vi "TLB Native Dynamic Events ver 0.04.vi"() -> ()   [LabVIEW 2018]
uses:
  Labview Training Phase 2/Enum Controls/States for Action Engine.ctl
  Type def/TLB event states.ctl
panel:
  out "element":T1
  in  "Combo Box":string(combo)
  in  "Stop Queue":bool
  in  "Start Queue":bool
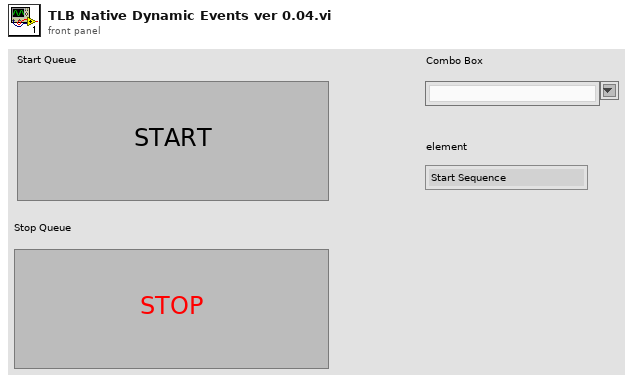
[diagram p1: front panel]
types:
  T1 = typedef "TLB event states.ctl" = enum16{"Start Sequence", "Exit", "Start Task 1", "Start Task 2", "Start Task 3", "Start Task 4", "Camera vision", "Wall follow mode", "Idle", "Start Drive Straight"}
  T2 = typedef "States for Action Engine.ctl" = enum16{"Initialize", "Write", "Read"}
  T3 = typedef "TLB event states.ctl" = enum16{"Start Sequence", "Exit", "Task 1", "Task 2"}
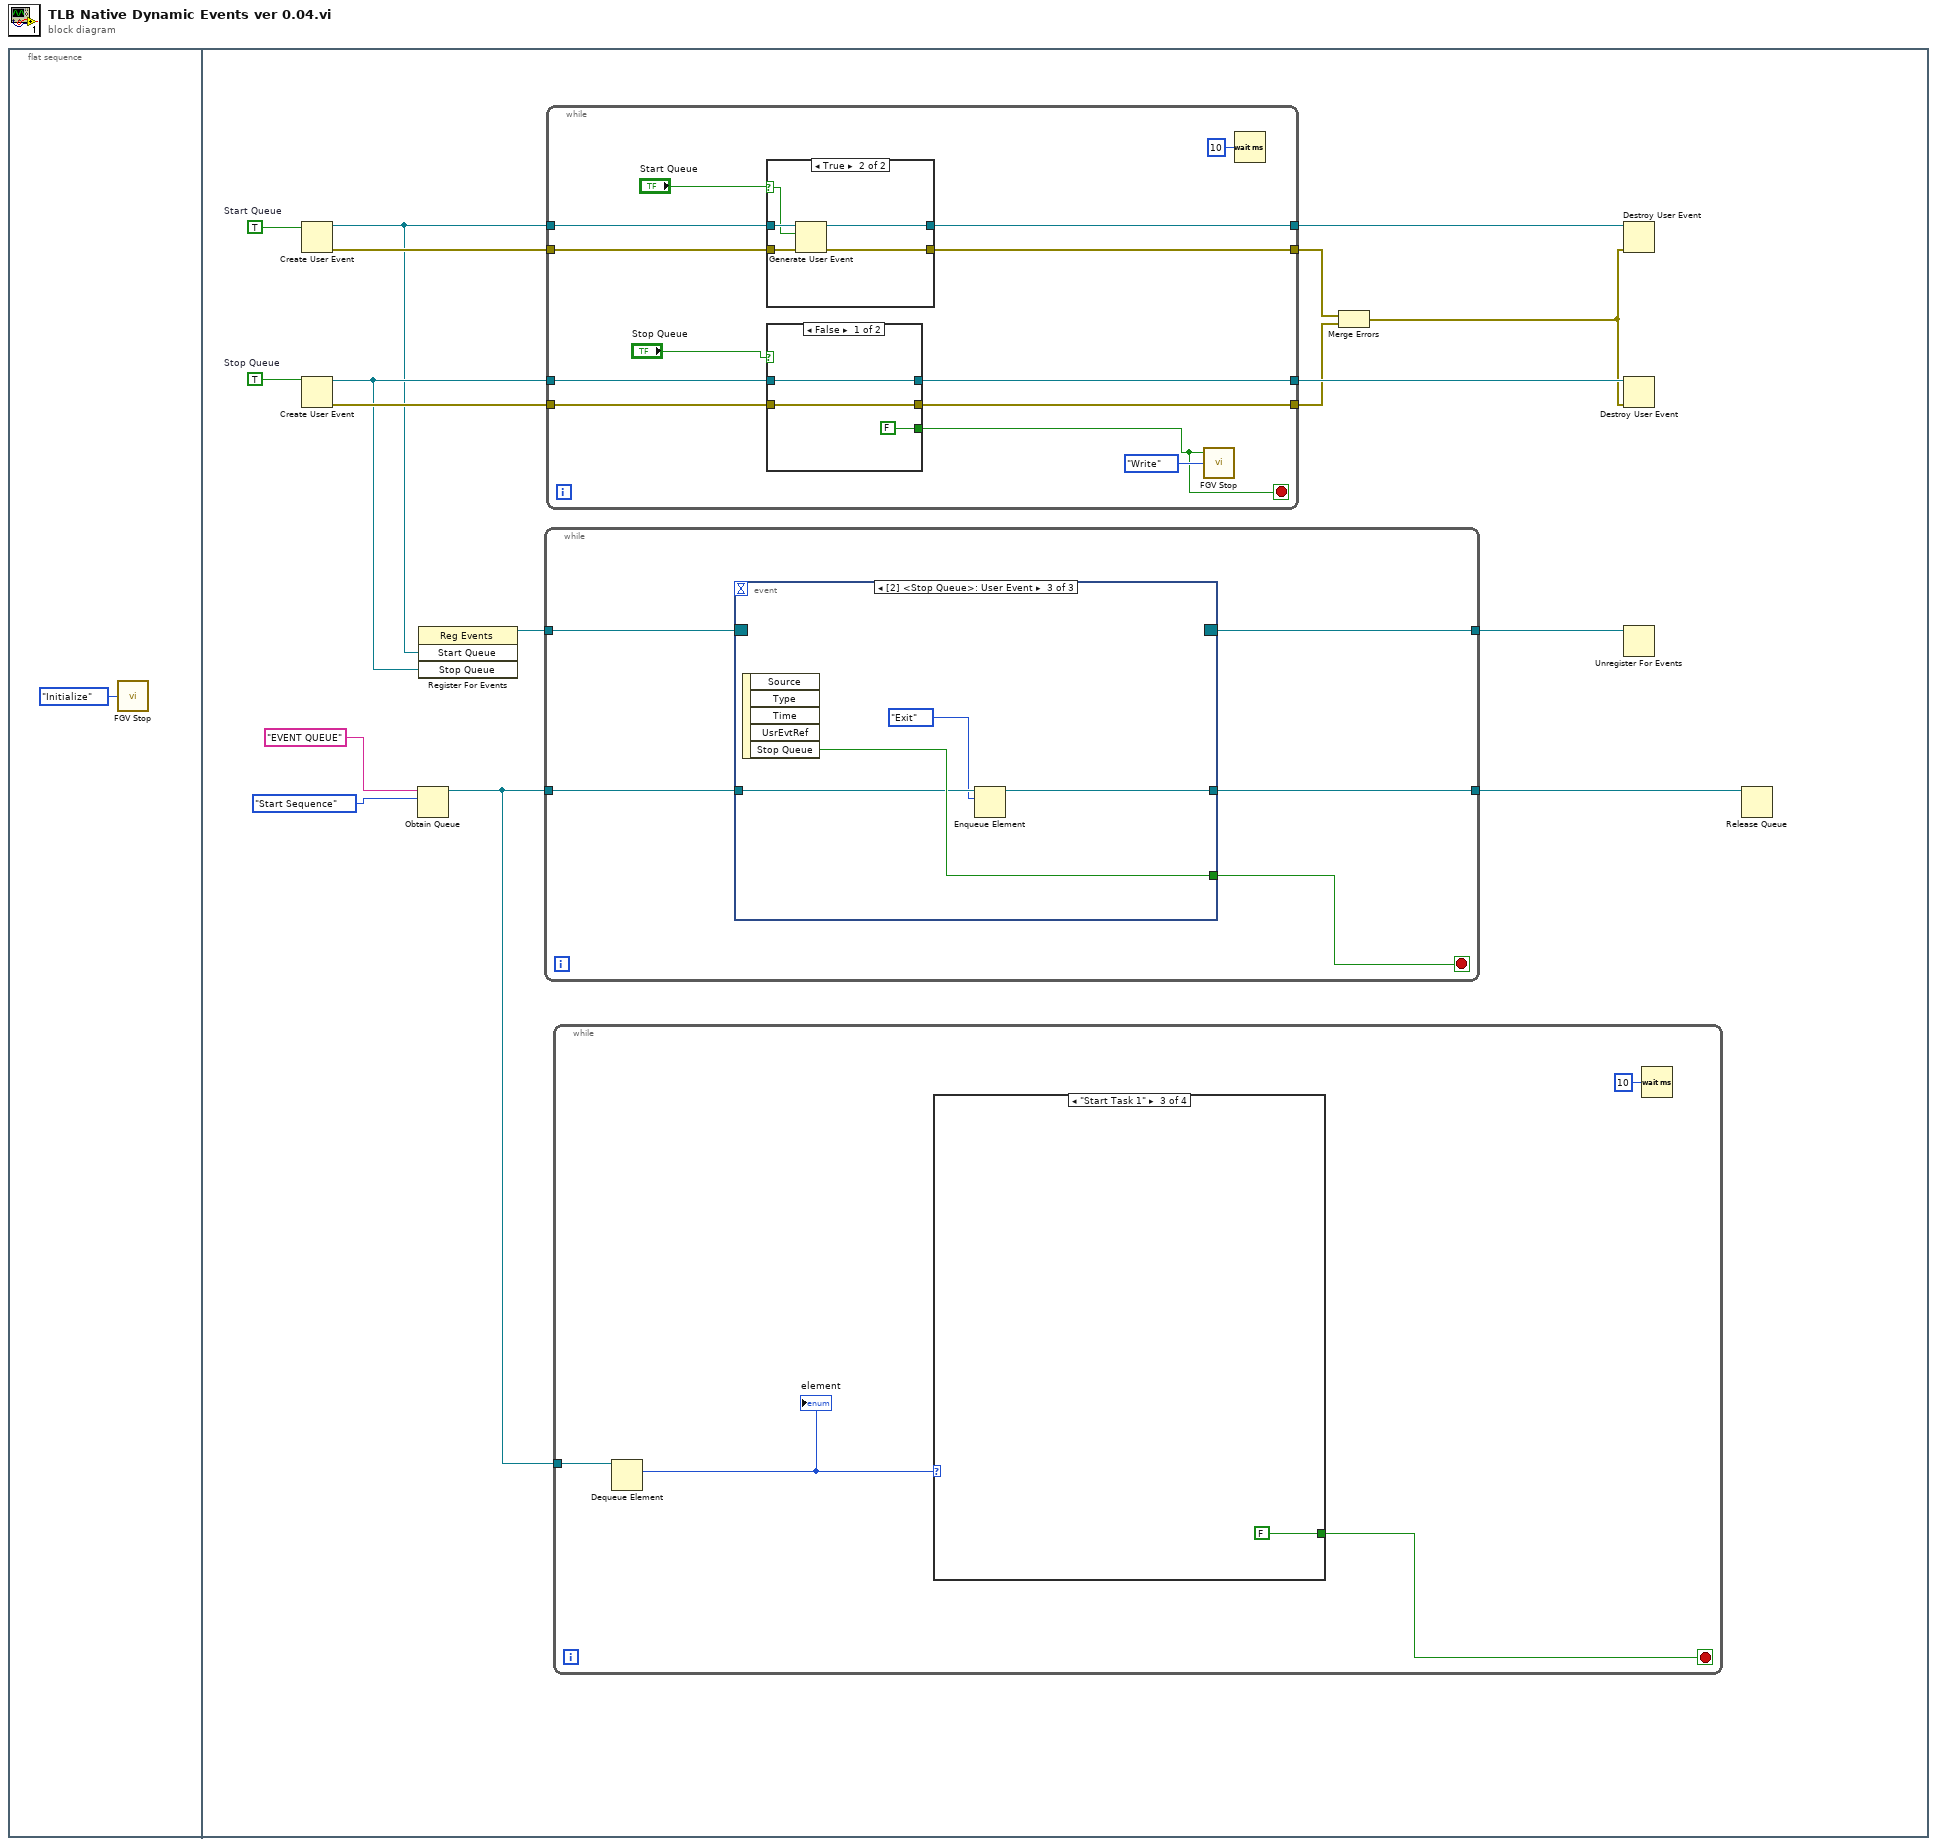
[diagram p0: block diagram]
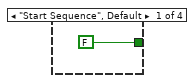
[diagram p2: hidden frame]
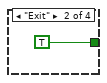
[diagram p3: hidden frame]
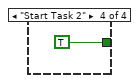
[diagram p4: hidden frame]
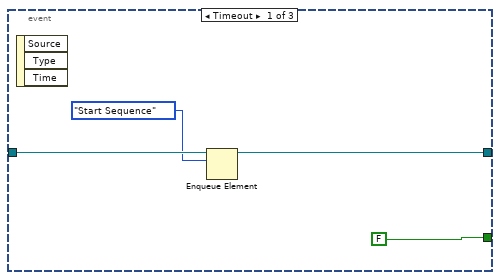
[diagram p5: hidden frame]
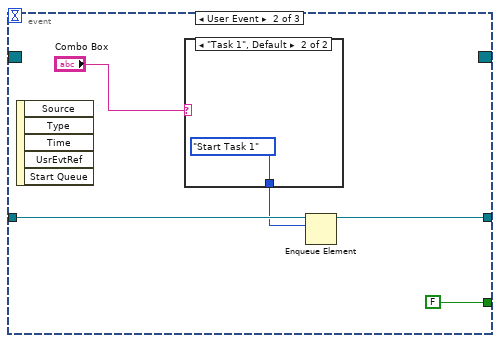
[diagram p6: hidden frame]
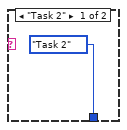
[diagram p7: hidden frame]
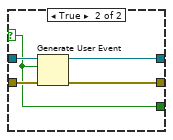
[diagram p8: hidden frame]
diagram:
  n1 = flat-sequence {
    frame #0 {
      n2 = call "FGV Stop.vi"("Init/Read/Write State"=States_for_Action_Engine."Initialize") -> ()  [unwired: 2 in, 2 out]
    }
    frame #1 {
      w18 = TRUE  # Stop Queue
      w17 = TRUE  # Start Queue
      n3 = Create User Event(user event datatype=w17) -> (user event=w8:refnum<user-event>, error out=w14:errorcluster)  [unwired: 1 in]
      n4 = Create User Event(user event datatype=w18) -> (user event=w9:refnum<user-event>, error out=w13:errorcluster)  [unwired: 1 in]
      n5 = Obtain Queue(name (unnamed)="EVENT QUEUE", element data type=TLB_event_states."Start Sequence" ("Enum")) -> (queue out=w2:refnum<queue>)  [unwired: 3 in, 2 out]
      n6 = register-events(w8, w9) -> (reference out=w7:refnum<event-registration>)  [unwired: 2 in, 1 out]
      n7 = while {
        tunnel: w7 -> [w31]
        tunnel: [w30] -> w6
        tunnel: w2 -> [w28]
        tunnel: [w27] -> w5
        stop <- w29 stop-if-true
        n8 = event shown="[2] <Stop Queue>: User Event" {
          selector: w31 -> [_ _ _]
          dyn-events: [_ _ _] -> w30
          timeout: _ -> [_ _ _]
          tunnel: [FALSE FALSE w46] -> w29
          tunnel: w28 -> [w34 w39 w44]
          tunnel: [w33 w38 w45] -> w27
          event Timeout {
            n9 = event-data() -> ()  [unwired: 1 in, 3 out]
            n10 = Enqueue Element(queue=w34, element=TLB_event_states."Start Sequence" ("Enum")) -> (queue out=w33:refnum<queue>)  [unwired: 2 in, 2 out]
          }
          event User Event {
            n11 = event-data() -> ()  [unwired: 1 in, 5 out]
            n12 = case shown="\"Task 1\", Default" "Combo Box" {
              tunnel: [TLB_event_states."Task 2" ("Enum") TLB_event_states."Start Task 1" ("Enum")] -> w36
              frame "Task 2" {
              }
              frame "Task 1", Default {
              }
            }
            n13 = Enqueue Element(queue=w39, element=w36) -> (queue out=w38:refnum<queue>)  [unwired: 2 in, 2 out]
          }
          event User Event {
            n14 = event-data() -> ("Stop Queue"=w46:bool)  [unwired: 1 in, 4 out]
            n15 = Enqueue Element(queue=w44, element=TLB_event_states."Exit" ("Enum")) -> (queue out=w45:refnum<queue>)  [unwired: 2 in, 2 out]
          }
        }
      }
      n16 = while {
        tunnel: w8 -> [w58]
        tunnel: w9 -> [w57]
        tunnel: [w56] -> w16
        tunnel: [w55] -> w15
        tunnel: w14 -> [w54]
        tunnel: [w53] -> w12
        tunnel: w13 -> [w52]
        tunnel: [w51] -> w11
        stop <- w47 stop-if-true
        n17 = case shown="True" "Start Queue" {
          selector: "Start Queue" -> [_ w70]
          tunnel: w58 -> [w69 w74]
          tunnel: [w69 w73] -> w55
          tunnel: w54 -> [w68 w72]
          tunnel: [w68 w71] -> w53
          frame False {
          }
          frame True {
            n18 = Generate User Event(user event=w74, event data cluster=w70, error in=w72) -> (user event out=w73:refnum<user-event>, error out=w71:errorcluster)  [unwired: 1 in]
          }
        }
        n19 = case shown="False" "Stop Queue" {
          selector: "Stop Queue" -> [_ w63]
          tunnel: w57 -> [w62 w67]
          tunnel: [w62 w66] -> w56
          tunnel: w52 -> [w61 w65]
          tunnel: [w61 w64] -> w51
          tunnel: [FALSE w63] -> w47
          frame False {
          }
          frame True {
            n20 = Generate User Event(user event=w67, event data cluster=w63, error in=w65) -> (user event out=w66:refnum<user-event>, error out=w64:errorcluster)  [unwired: 1 in]
          }
        }
        n21 = call "FGV Stop.vi"("Init/Read/Write State"=States_for_Action_Engine."Write", "Input Node"=w47) -> ()  [unwired: 1 in, 2 out]
        n22 = Wait (ms)(milliseconds to wait=u32 10) -> ()  [unwired: 1 out]
      }
      n23 = while {
        tunnel: w2 -> [w21]
        stop <- w19 stop-if-true
        n24 = Dequeue Element(queue=w21) -> (element=w20:T1)  [unwired: 2 in, 3 out]
        "element" <- w20
        n25 = case shown="\"Start Task 1\"" w20 {
          tunnel: [FALSE TRUE FALSE TRUE] -> w19
          frame "Start Sequence", Default {
          }
          frame "Exit" {
          }
          frame "Start Task 1" {
          }
          frame "Start Task 2" {
          }
        }
        n26 = Wait (ms)(milliseconds to wait=u32 10) -> ()  [unwired: 1 out]
      }
      n27 = Merge Errors(w12, w11) -> (w10:errorcluster)
      n28 = Destroy User Event(user event=w15, error in=w10) -> ()  [unwired: 1 out]
      n29 = Destroy User Event(user event=w16, error in=w10) -> ()  [unwired: 1 out]
      n30 = Unregister For Events(event registration refnum=w6) -> ()  [unwired: 1 in, 1 out]
      n31 = Release Queue(queue=w5) -> ()  [unwired: 2 in, 3 out]
    }
  }
